vi "FSK 1 bits.vi"() -> ()   [LabVIEW 2010]
panel:
  out "Demodulation":dynamicdata(graph)
  out "Valeur Comparaison":dynamicdata(graph)
  out "Modulation":dynamicdata(graph)
  in  "Tableau":bool[](array[boolean])
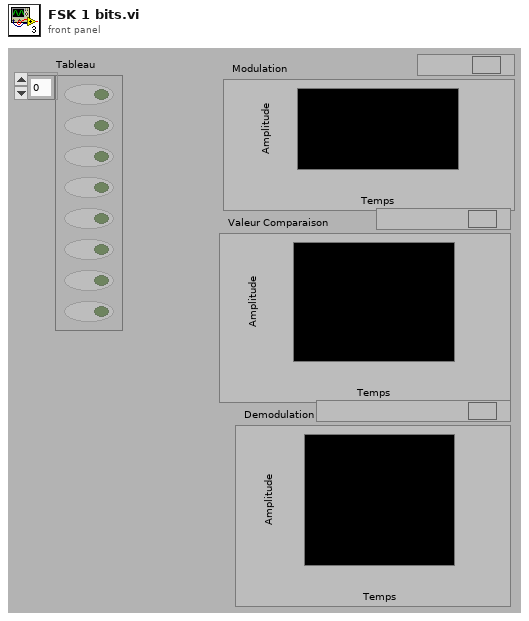
[diagram p1: front panel]
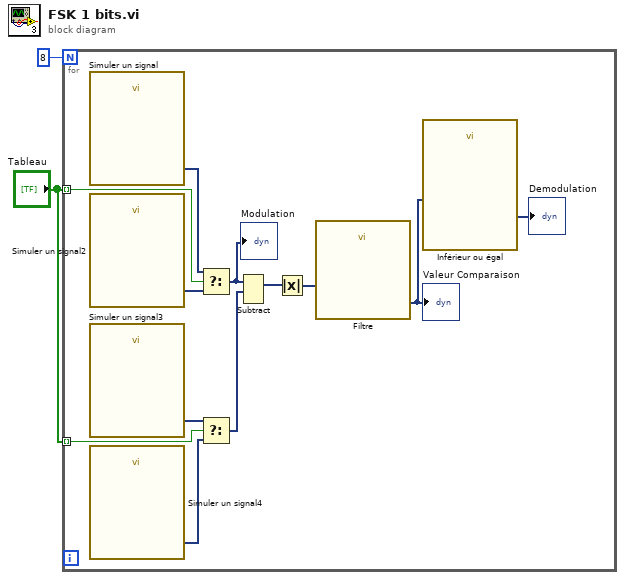
[diagram p0: block diagram]
diagram:
  n1 = for {
    N: 8 -> [_]
    tunnel: "Tableau" -> [w14] mode=indexing
    tunnel: "Tableau" -> [w13] mode=indexing
    n2 = call "Simuler un signal"() -> ("Sinus"=w12:dynamicdata)  [unwired: 14 in, 1 out]
    n3 = call "Simuler un signal2"() -> ("Sinus"=w11:dynamicdata)  [unwired: 14 in, 1 out]
    n4 = call "Simuler un signal3"() -> ("Sinus"=w10:dynamicdata)  [unwired: 14 in, 1 out]
    n5 = call "Simuler un signal4"() -> ("Sinus"=w9:dynamicdata)  [unwired: 14 in, 1 out]
    n6 = Select(t=w12, s=w14, f=w11) -> (s? t:f=w6:dynamicdata)
    "Modulation" <- w6
    n7 = Select(t=w10, s=w13, f=w9) -> (s? t:f=w8:dynamicdata)
    n8 = Subtract(1:w8, 2:w6) -> (0:w7:dynamicdata)  [unwired: 1 in, 1 out]
    n9 = Absolute Value(x=w7) -> (abs(x)=w5:dynamicdata)
    n10 = call "Filtre"("Signal"=w5) -> ("Filtered Signal"=w4:dynamicdata)  [unwired: 9 in, 1 out]
    "Valeur Comparaison" <- w4
    n11 = call "Inférieur ou égal"("Operand 1"=w4) -> ("Result"=→"Demodulation":dynamicdata)  [unwired: 9 in, 1 out]
  }
